vi "RX-FIR2.vi"() -> ()   [LabVIEW 2019]
uses:
  <vilib>/sound2/lvsound2.llb/Sound Data Format.ctl
  <instrlib>/niUSRP/niUSRP Fetch Rx Data (CDB WDT).vi
  <vilib>/Analysis/3filter.llb/FIR Filter (DBL).vi
  <vilib>/Analysis/2dsp.llb/Rational Resample (single channel, DBL).vi
  <vilib>/express/express analysis/Spectral/Block/exnSpectralBlock spectral measurements RMS poly.vi
  <vilib>/express/express analysis/Spectral/Block/exnSpectralBlock spectral measurements RMS WFM.vi
  <vilib>/sound2/lvsound2.llb/Sound Output Write (DBL Single).vi
  <vilib>/express/express analysis/Spectral/XNode/ExpressSpectralMeasurementsBlockNode.xnode
  <vilib>/Analysis/NI_AALPro.lvlib
  <vilib>/Analysis/NI_AALBase.lvlib
panel:
  out "error out 2":errorcluster
  in  "sound format":T1={"sample rate (S/s)"=44100.0, "number of channels"=1, "bits per sample"=16}
  in  "number of samples":i64=44100
  out "coerced gain":dbl format="%#_6f"
  out "coerced carrier frequency":dbl=2400000000.0 format="%#_6p"
  out "coerced IQ rate":dbl=200000.0 format="%#_6p"
  in  "active antenna":string="RX2"
  in  "gain":dbl format="%#_6f"
  in  "carrier frequency":dbl=2400000000.0 format="%#_6p"
  in  "IQ rate":dbl=200000.0 format="%#_6p"
  out "error out":errorcluster
  in  "device names":refnum<k15>="192.168.10.4"
  in  "stop":bool
  out "Waveform Graph":cluster{"f0":dbl, "df":dbl, "magnitude":dbl[]}(graph)
  out "XY Graph":cluster{dbl[], dbl[]}(graph)
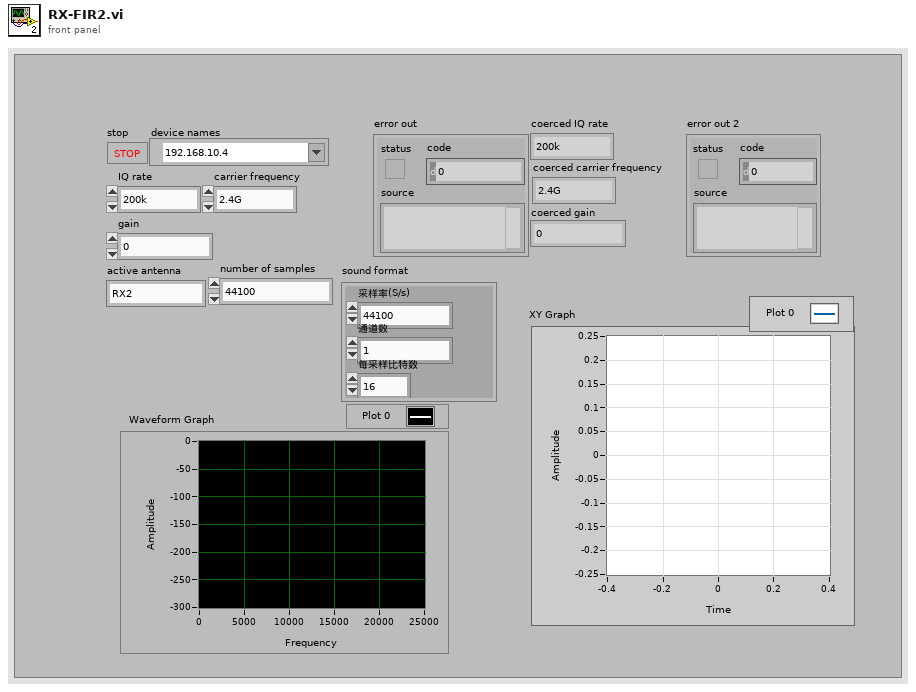
[diagram p1: front panel]
types:
  T1 = typedef "Sound Data Format.ctl" = cluster{"sample rate (S/s)":dbl, "number of channels":i32, "bits per sample":i32}
  T2 = typedef "Sound Output Task ID.ctl" = u32
  T3 = cluster{"averaging mode":u16, "weighting mode":u16, "number of averages":u32}
  T4 = cluster{"dB On (F)":bool, "unwrap phase (F)":bool, "convert to degree (F)":bool}
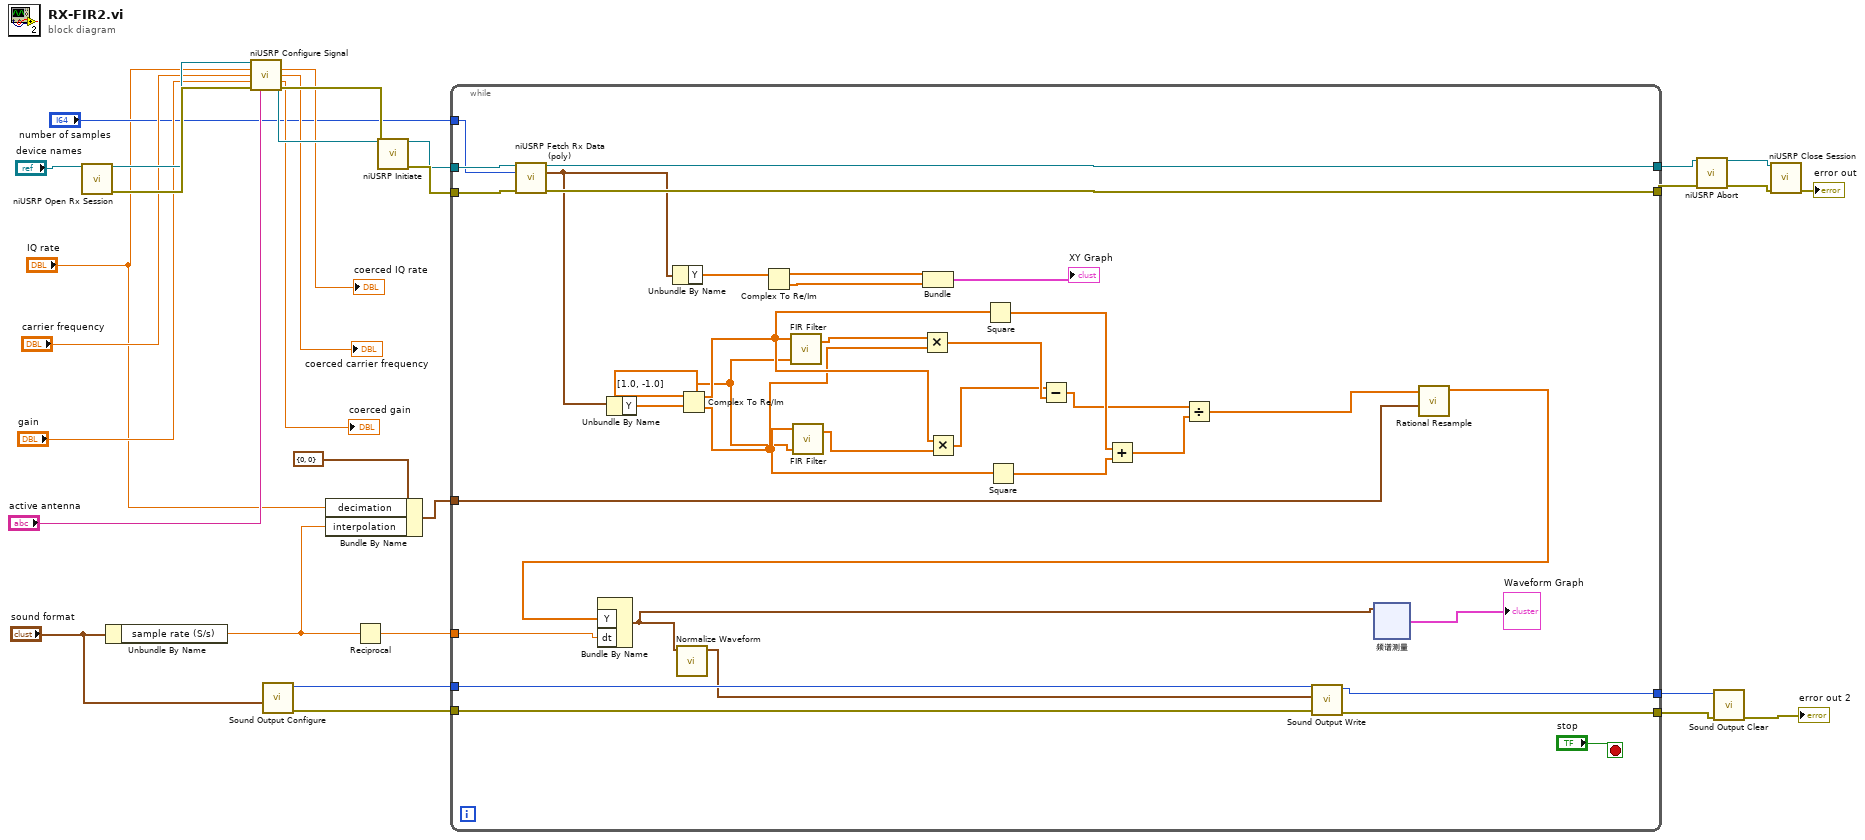
[diagram p0: block diagram]
diagram:
  n1 = call <instrlib>:"niUSRP Open Rx Session.vi"("device names"="device names") -> ("session handle out"=w19:refnum<k15>, "error out"=w29:errorcluster)  [unwired: 13 in]
  n2 = Unbundle By Name("sound format") -> ("sample rate (S/s)"=w9:dbl)
  n3 = call <instrlib>:"niUSRP Configure Signal.vi"("session handle"=w19, "IQ rate"="IQ rate", "carrier frequency"="carrier frequency", "gain"="gain", "error in (no error)"=w29, "active antenna"="active antenna") -> ("session handle out"=w20:refnum<k15>, "coerced IQ rate"=→"coerced IQ rate":dbl, "coerced carrier frequency"=→"coerced carrier frequency":dbl, "coerced gain"=→"coerced gain":dbl, "error out"=w28:errorcluster)  [unwired: 5 in]
  n4 = call <vilib>:"Sound Output Configure.vi"("sound format"="sound format") -> ("error out"=w8:errorcluster, "task ID"=w3:T2)  [unwired: 9 in]
  n5 = Bundle By Name(cluster=cluster{"decimation":i32, "interpolation":i32} {"decimation"=0, "interpolation"=0}, "decimation"="IQ rate", "interpolation"=w9) -> (w4:cluster{"decimation":i32, "interpolation":i32})
  n6 = Reciprocal(x=w9) -> (1/x=w5:dbl)
  n7 = call <instrlib>:"niUSRP Initiate.vi"("session handle"=w20, "error in (no error)"=w28) -> ("session handle out"=w23:refnum<k15>, "error out"=w27:errorcluster)  [unwired: 12 in]
  n8 = while {
    tunnel: w27 -> [w63]
    tunnel: [w62] -> w26
    tunnel: w23 -> [w61]
    tunnel: [w60] -> w22
    tunnel: "number of samples" -> [w59]
    tunnel: w8 -> [w58]
    tunnel: [w57] -> w7
    tunnel: w5 -> [w56]
    tunnel: w4 -> [w55]
    tunnel: w3 -> [w53]
    tunnel: [w52] -> w2
    stop <- "stop" stop-if-true
    w31 = dbl[] [1.0, -1.0] ("FIR Coefficients")
    n9 = call-poly <instrlib>:"niUSRP Fetch Rx Data (poly).vi"("session handle"=w61, "number of samples"=w59, "error in (no error)"=w63) -> ("session handle out"=w60:refnum<k15>, "data"=w44:waveform(cdb), "error out"=w62:errorcluster)  [unwired: 9 in, 1 out]
    n10 = Unbundle By Name(w44) -> ("Y"=w43:cdb[])
    n11 = Unbundle By Name(w44) -> ("Y"=w48:cdb[])
    n12 = Complex To Re/Im(x + iy=w43) -> (x=w40:dbl[], y=w32:dbl[])
    n13 = Complex To Re/Im(x + iy=w48) -> (x=w47:dbl[], y=w46:dbl[])
    n14 = call-poly <vilib>:"FIR Filter.vi"("FIR Coefficients"=w31, "X"=w40) -> ("Filtered X"=w42:dbl[])  [unwired: 2 in, 1 out]
    n15 = call-poly <vilib>:"FIR Filter.vi"("FIR Coefficients"=w31, "X"=w32) -> ("Filtered X"=w41:dbl[])  [unwired: 2 in, 1 out]
    n16 = Multiply(x=w42, y=w32) -> (x*y=w39:dbl[])
    n17 = Bundle(w47, w46) -> (→"XY Graph":cluster{dbl[], dbl[]})  [unwired: 1 in]
    n18 = Multiply(x=w40, y=w41) -> (x*y=w38:dbl[])
    n19 = Square(x=w40) -> (x^2=w36:dbl[])
    n20 = Square(x=w32) -> (x^2=w37:dbl[])
    n21 = Subtract(x=w38, y=w39) -> (x-y=w35:dbl[])
    n22 = Add(x=w36, y=w37) -> (x+y=w34:dbl[])
    n23 = Divide(x=w35, y=w34) -> (x/y=w33:dbl[])
    n24 = call-poly <vilib>:"Rational Resample.vi"("resample factor"=w55, "X"=w33) -> ("Y"=w54:dbl[])  [unwired: 7 in, 2 out]
    n25 = Bundle By Name("Y"=w54, "dt"=w56) -> (w50:waveform(dbl))  [unwired: 1 in]
    n26 = call <vilib>:"Normalize Waveform.vi"("waveform in"=w50) -> ("normalized waveform"=w51:waveform(dbl))  [unwired: 7 in, 3 out]
    n27 = call-poly <vilib>:"Sound Output Write.vi"("error in (no error)"=w58, "data"=w51, "task ID"=w53) -> ("error out"=w57:errorcluster, "task ID out"=w52:T2)  [unwired: 7 in]
    n28 = xnode ("频谱测量")("信号"=w50) -> ("FFT - (RMS)"=→"Waveform Graph":cluster{"f0":dbl, "df":dbl, "magnitude":dbl[]})  [unwired: 1 in, 2 out]
  }
  n29 = call <instrlib>:"niUSRP Abort.vi"("session handle"=w22, "error in (no error)"=w26) -> ("session handle out"=w21:refnum<k15>, "error out"=w25:errorcluster)  [unwired: 12 in]
  n30 = call <vilib>:"Sound Output Clear.vi"("error in (no error)"=w7, "task ID"=w2) -> ("error out"=→"error out 2":errorcluster)  [unwired: 9 in]
  n31 = call <instrlib>:"niUSRP Close Session.vi"("session handle"=w21, "error in (no error)"=w25) -> ("error out"=→"error out":errorcluster)  [unwired: 13 in]
